vi "Error to Dialogue Message.vi"(1 "error in":errorcluster) -> (0 "Dialogue Message":string)   [LabVIEW 2020]
doc: "Raises a custom, user-generated error if and only if there is no error at the \"error in\" input.\n\nIn other words, this VI does not overwrite an existing error. This behaviour is believed to be desirable in most cases."
panel:
  # "Development\ncontrols/indicators useful for development and testing, but which are not outputs of the VI"
  # "Input\nInputs to the VI"
  # "Output\nOutputs of the VI"
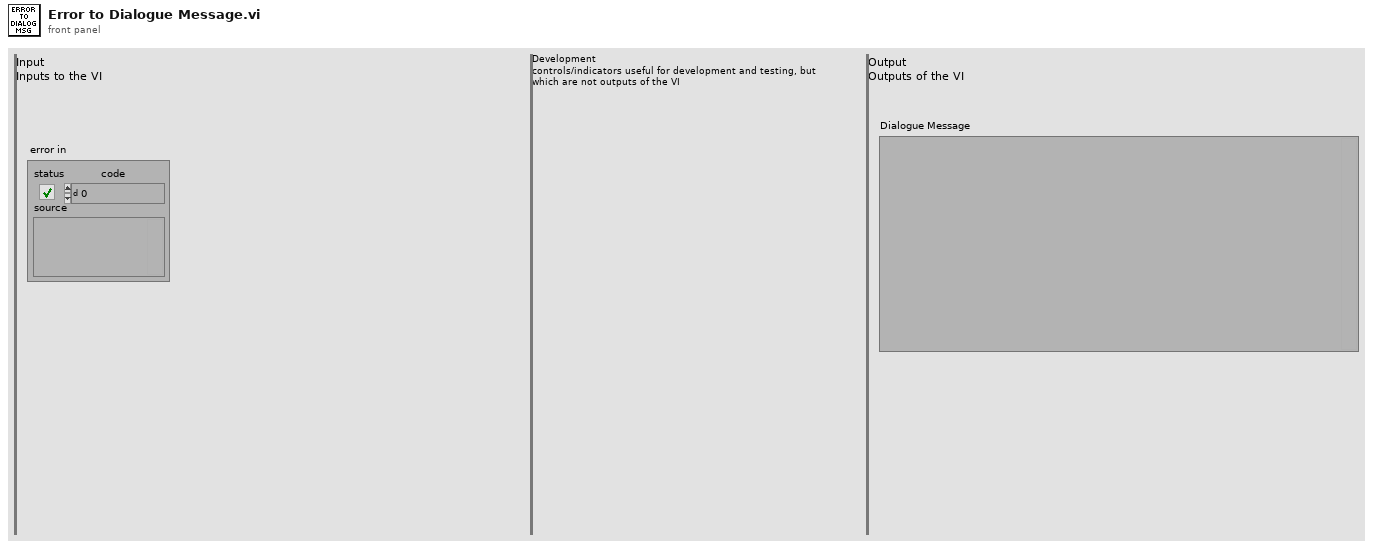
[diagram p1: front panel]
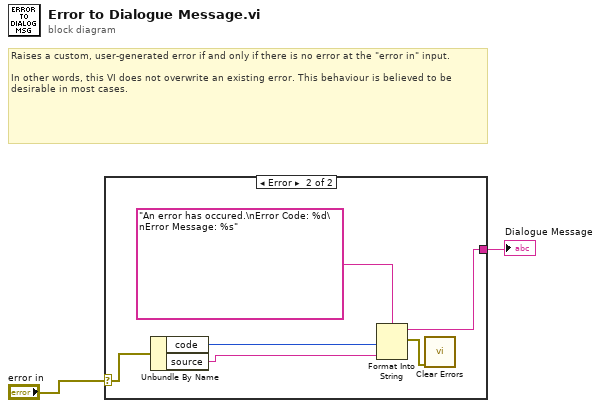
[diagram p0: block diagram]
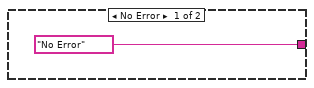
[diagram p2: hidden frame]
diagram:
  # "Raises a custom, user-generated error if and only if there is no error at the \"error in\" input.\n\nIn other words, this VI does not overwrite an existing error. This behaviour is believed to be desirable in most cases."
  n1 = case shown="Error" "error in" {
    selector: "error in" -> [_ w6]
    tunnel: ["No Error" w8] -> w1
    frame No Error {
    }
    frame Error {
      n2 = Unbundle By Name(w6) -> ("code"=w5:i32, "source"=w4:string)
      n3 = Format Into String(format string="An error has occured.\nError Code: %d\nError Message: %s", w5, w4) -> (resulting string=w8:string, error out=w7:errorcluster)  [unwired: 2 in]
      n4 = call <vilib>:"Clear Errors.vi"("error in (no error)"=w7) -> ()  [unwired: 5 in, 2 out]
    }
  }
  "Dialogue Message" <- w1
